vi "Update Elevator Position.vi"(8 "error in (no error)":errorcluster, 10 "Elevator Position":u8, 11 "Sim Sensor Interface Actor in":refnum<class "Sim Sensor Interface Actor.lvclass">) -> (0 "error out":errorcluster, 3 "Sim Sensor Interface Actor out":refnum<class "Sim Sensor Interface Actor.lvclass">)   [LabVIEW 2022 SP3, in "Sim Sensor Interface Actor.lvlib" / "Sim Sensor Interface Actor.lvclass"]
uses:
  Sim Sensor Interface Actor.lvclass
  Sim Sensor Interface Actor.lvclass/Sim Sensor Interface Actor.ctl
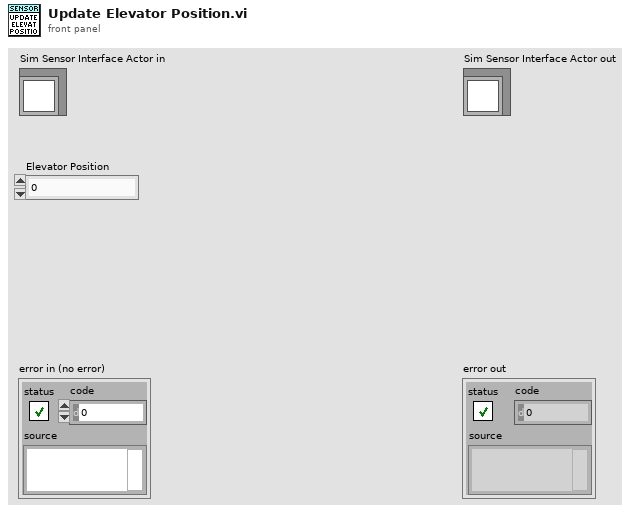
[diagram p1: front panel]
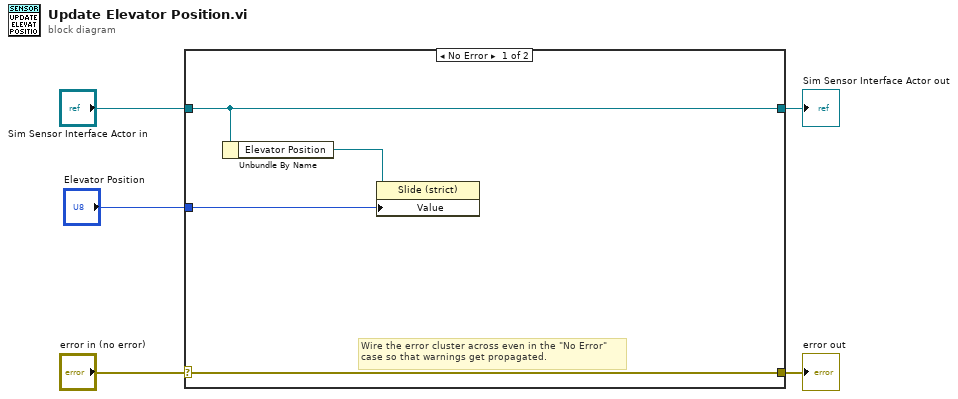
[diagram p0: block diagram]
diagram:
  n1 = case shown="No Error" "error in (no error)" {
    selector: "error in (no error)" -> [w9 w11]
    tunnel: [w9 w11] -> w4
    tunnel: [w8 w10] -> w2
    tunnel: "Sim Sensor Interface Actor in" -> [w8 w10]
    tunnel: "Elevator Position" -> [w6 _]
    frame No Error {
      # "Wire the error cluster across even in the \"No Error\"\ncase so that warnings get propagated."
      n2 = Unbundle By Name(w8) -> ("Elevator Position"=w7:refnum<vi>)
      n3 = property class="Slide (strict)"(reference=w7, "Value"=w6) -> ()  [unwired: 1 in, 2 out]
    }
    frame Error {
    }
  }
  "error out" <- w4
  "Sim Sensor Interface Actor out" <- w2
